vi "Math-Moving Average.vi"(9 "Iterations":i32, 10 "Length":i32, 11 "Array in":dbl[](array[numeric])) -> (3 "Array out":dbl[](array[numeric]))   [LabVIEW 2020]
uses:
  <vilib>/Analysis/2dsp.llb/1D Convolution (DBL).vi
  <vilib>/Analysis/NI_AALPro.lvlib
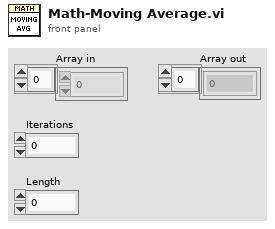
[diagram p1: front panel]
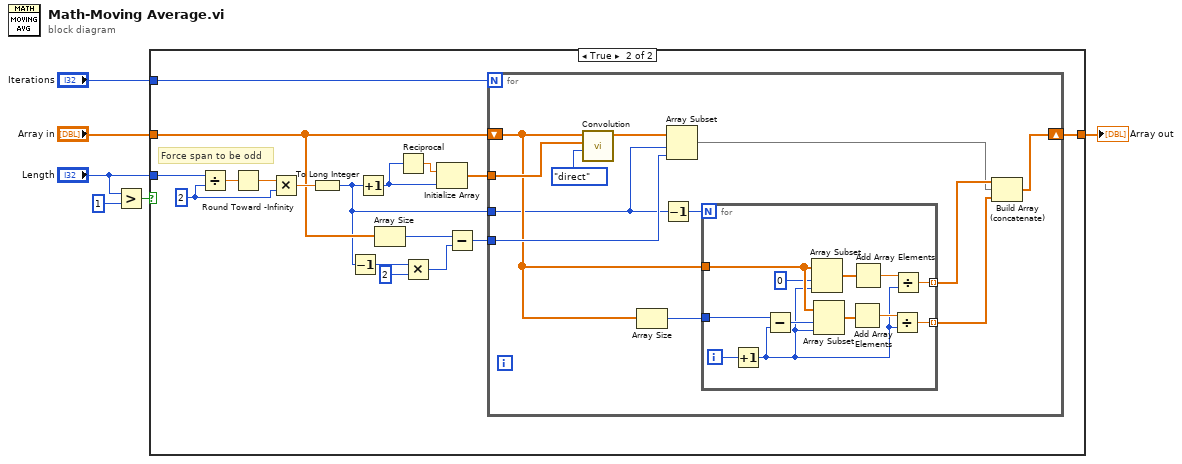
[diagram p0: block diagram]
diagram:
  n1 = Greater?(x="Length", y=1 ("x")) -> (0:w3:bool)
  n2 = case shown="True" w3 {
    tunnel: [w7 w24] -> w6
    tunnel: "Iterations" -> [_ w22]
    tunnel: "Length" -> [_ w17]
    tunnel: "Array in" -> [w7 w16]
    frame False {
    }
    frame True {
      w19 = 2 ("y")
      # "Force span to be odd"
      n3 = Divide(x=w17, y=w19) -> (x/y=w20:dbl)
      n4 = Round Toward -Infinity(1:w20) -> (0:w13:dbl)
      n5 = Multiply(x=w13, y=w19) -> (x*y=w18:dbl)
      n6 = To Long Integer(number=w18) -> (32bit integer=w12:i32)
      n7 = Decrement(x=w12) -> (x-1=w8:i32)
      n8 = Increment(x=w12) -> (x+1=w9:i32)
      n9 = Array Size(array=w16) -> (size(s)=w15:i32)
      n10 = Reciprocal(x=w9) -> (1/x=w21:dbl)
      n11 = Multiply(x=w8, y=2) -> (x*y=w11:i32)
      n12 = Initialize Array(w21, w9) -> (w23:dbl[])
      n13 = Subtract(x=w15, y=w11) -> (x-y=w14:i32)
      n14 = for {
        N: w22 -> [_]
        tunnel: w23 -> [w36]
        shift-right: [w30] -> w24
        shift-left: w16 -> [w28]
        tunnel: w12 -> [w26]
        tunnel: w14 -> [w34]
        n15 = call-poly <vilib>:"Convolution.vi"("algorithm"=enum32{"direct", "frequency domain"}."direct", "Y"=w36, "X"=w28) -> ("X * Y"=w35:dbl[])  [unwired: 7 in, 1 out]
        n16 = Array Size(array=w28) -> (size(s)=w27:i32)
        n17 = Decrement(x=w26) -> (x-1=w25:i32)
        n18 = Array Subset(array=w35, index=w26, length=w34) -> (w31:dbl[])
        n19 = for {
          N: w25 -> [_]
          tunnel: w28 -> [w45]
          tunnel: [w46] -> w32 mode=indexing
          tunnel: [w42] -> w29 mode=indexing
          tunnel: w27 -> [w41]
          i -> [w40]
          n20 = Increment(x=w40) -> (x+1=w38:i32)
          n21 = Subtract(x=w41, y=w38) -> (x-y=w39:i32)
          n22 = Array Subset(array=w45, index=0, length=w38) -> (w47:dbl[])
          n23 = Array Subset(array=w45, index=w39, length=w38) -> (w43:dbl[])
          n24 = Add Array Elements(numeric array=w43) -> (sum=w44:dbl)
          n25 = Add Array Elements(numeric array=w47) -> (sum=w48:dbl)
          n26 = Divide(x=w44, y=w38) -> (x/y=w42:dbl)
          n27 = Divide(x=w48, y=w38) -> (x/y=w46:dbl)
        }
        n28 = Build Array (concatenate)(w32, w31, w29) -> (w30:dbl[])
      }
    }
  }
  "Array out" <- w6
